vi "Sort Impulses.vi"(8 "error in (no error)":errorcluster, 9 "Impulse Select":T1, 10 "Impulse Positions":T2(array[cluster]) {"Amplitude offset" format="%.2f"}, 11 "Data Input":T3 {"Data Channels" format="%.2f"}) -> (0 "error out":errorcluster, 1 "Num Impulses":i32, 2 "Impulses Duration (samples)":i32, 3 "Impulse Data":dbl[][](array[numeric]), 5 "Channel Index":i32[](array[numeric]))   [LabVIEW 2016]
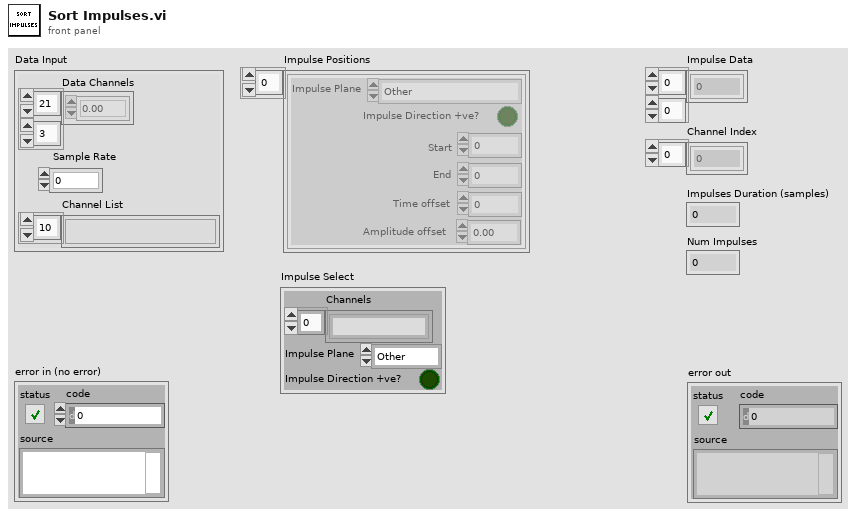
[diagram p1: front panel]
types:
  T1 = cluster{"Channels":string[], "Impulse Plane":enum16{"Other", "Yaw", "Pitch", "Roll", "LARP", "RALP"}, "Impulse Direction +ve?":bool}
  T2 = cluster{"Start":i32, "End":i32, "Impulse Plane":enum16{"Other", "Yaw", "Pitch", "Roll", "LARP", "RALP"}, "Impulse Direction +ve?":bool, "Time offset":i32, "Amplitude offset":dbl}[]
  T3 = cluster{"Data Channels":dbl[][], "Sample Rate":i32, "Channel List":string[]}
  T4 = enum16{"Other", "Yaw", "Pitch", "Roll", "LARP", "RALP"}
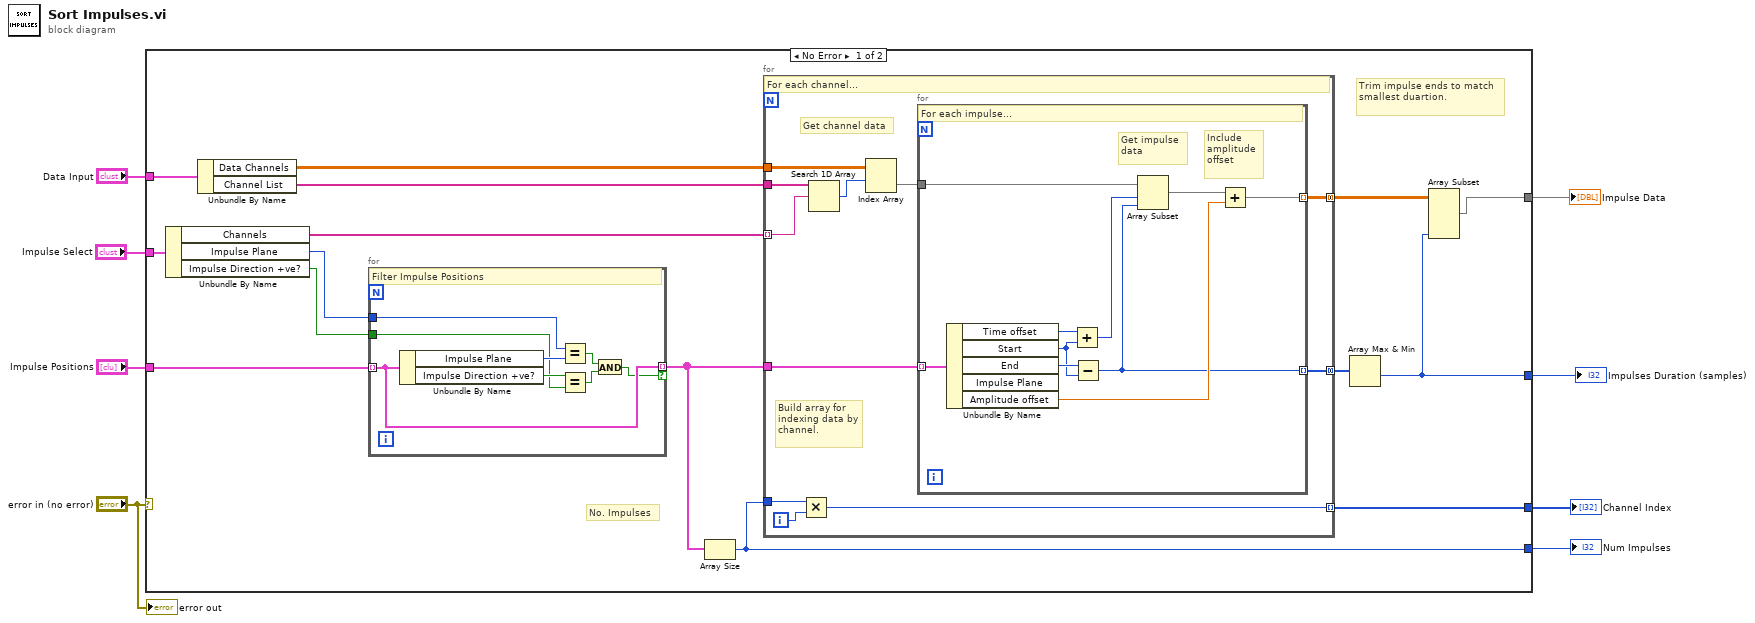
[diagram p0: block diagram]
diagram:
  n1 = case shown="No Error" "error in (no error)" {
    tunnel: "Data Input" -> [w23 _]
    tunnel: "Impulse Positions" -> [w18 _]
    tunnel: "Impulse Select" -> [w20 _]
    tunnel: [w10 _] -> w6
    tunnel: [w14 _] -> w4
    tunnel: [w13 _] -> w2
    tunnel: [w9 _] -> w1
    frame No Error {
      # "Trim impulse ends to match smallest duartion."
      # "No. Impulses"
      n2 = Unbundle By Name(w20) -> ("Channels"=w19:string[], "Impulse Plane"=w17:T4, "Impulse Direction +ve?"=w16:bool)
      n3 = Unbundle By Name(w23) -> ("Data Channels"=w21:dbl[][], "Channel List"=w22:string[])
      n4 = for {
        tunnel: w18 -> [w25] mode=indexing
        tunnel: w17 -> [w30]
        tunnel: w16 -> [w28]
        tunnel: [w25] -> w15 mode=indexing if=w24
        # "Filter Impulse Positions"
        n5 = Unbundle By Name(w25) -> ("Impulse Plane"=w31:T4, "Impulse Direction +ve?"=w29:bool)
        n6 = Equal?(x=w30, y=w31) -> (x = y?=w27:bool)
        n7 = Equal?(x=w29, y=w28) -> (x = y?=w26:bool)
        n8 = And(x=w27, y=w26) -> (x .and. y?=w24:bool)
      }
      n9 = Array Size(array=w15) -> (size(s)=w14:i32)
      n10 = for {
        tunnel: w19 -> [w41] mode=indexing
        tunnel: w22 -> [w42]
        tunnel: w21 -> [w40]
        tunnel: [w37] -> w11 mode=concatenating
        tunnel: w15 -> [w36]
        tunnel: w14 -> [w34]
        tunnel: [w33] -> w13 mode=indexing
        tunnel: [w32] -> w12 mode=concatenating
        i -> [w35]
        # "Build array for indexing data by channel."
        # "Get channel data"
        # "For each channel..."
        n11 = Multiply(x=w34, y=w35) -> (x*y=w33:i32)
        n12 = Search 1D Array(1D array=w42, element=w41) -> (index of element=w39:i32)  [unwired: 1 in]
        n13 = Index Array(array=w40, index (row)=w39) -> (element=w38:dbl[])  [unwired: 1 in]
        n14 = for {
          tunnel: w38 -> [w51]
          tunnel: w36 -> [w52] mode=indexing
          tunnel: [w44] -> w37 mode=indexing
          tunnel: [w43] -> w32 mode=indexing
          # "Include amplitude offset"
          # "Get impulse data"
          # "For each impulse..."
          n15 = Unbundle By Name(w52) -> ("Time offset"=w50:i32, "Start"=w48:i32, "End"=w49:i32, "Amplitude offset"=w45:dbl)  [unwired: 1 out]
          n16 = Add(x=w50, y=w48) -> (x+y=w47:i32)
          n17 = Subtract(x=w49, y=w48) -> (x-y=w43:i32)
          n18 = Array Subset(array=w51, index=w47, length=w43) -> (w46:dbl[])
          n19 = Add(x=w46, y=w45) -> (x+y=w44:dbl[])
        }
      }
      n20 = Array Max & Min(array=w12) -> (min value=w9:i32)  [unwired: 3 out]
      n21 = Array Subset(array=w11, length (col)=w9) -> (w10:dbl[][])  [unwired: 3 in]
    }
    frame Error {
    }
  }
  "Impulse Data" <- w6
  "Channel Index" <- w2
  "Num Impulses" <- w4
  "Impulses Duration (samples)" <- w1
  "error out" <- "error in (no error)"
